vi "GotoWaypoint.vi"(7 "InhibitIn":bool, 8 "CurrentSteerAngle":dbl, 9 "WhatAroundMe? Clean":cluster{"T":dbl, "Range":dbl, "Bearing":dbl}[](array[cluster]), 10 "WhereAmI? Clean":T3, 11 "MDF In":T2(array[cluster])) -> (0 "BehCom":T1(ring), 1 "MDF Out":T2(array[cluster]), 2 "ActCommand":dbl[](array[numeric]), 4 "InhibitOut":bool, 5 "Vel":dbl, 6 "SteerAngle":dbl)   [LabVIEW 2012]
doc: "This subVI contains the Forebrain Goto Waypoint behaviors. Its inputs are the outputs of thewhat and where SENSE processes, theMission efinition Filet, a suppression value from another co-brahvior and an inhibit signal to turn the behavior off. The outputs are a 90 element steering array and a suppression value to diminish the output of co-behaviors.\n\nIt is designed to work with a 90 element behavior arbiter."
uses:
  <vilib>/Analysis/1siggen.llb/Ramp Pattern by Samples.vi
  <vilib>/gmath/statdist.llb/Normal PDF.vi
  <vilib>/gmath/NI_Gmath.lvlib
  <vilib>/Analysis/NI_AALBase.lvlib
panel:
  out "loop index":i32
  in  "HowAmI? Clean":cluster{"T":dbl, "Battery":dbl, "Temp":dbl}
  # "This VI contains the go to waypoint behavior  at the Forebrain level"
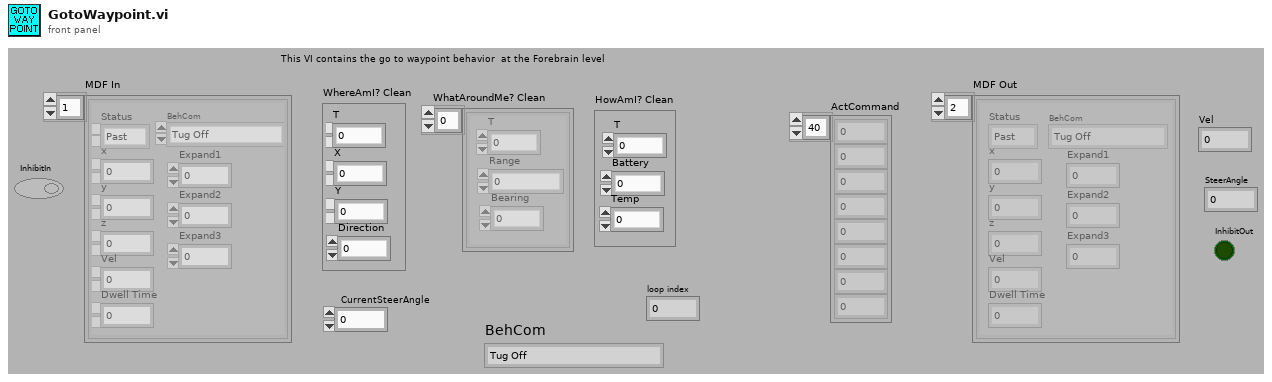
[diagram p1: front panel]
types:
  T1 = enum16{"Tug Off", "Manual Mode", "Goto WayPoint", "Back Up", "Circle", "Left Wall Follow", "Right Wall Follow", "Hunt"}
  T2 = cluster{"Status":enum16{"Past", "Current", "Future"}, "x":dbl, "y":dbl, "z":dbl, "Vel":dbl, "Dwell Time":dbl, "BehCom":enum16{"Tug Off", "Manual Mode", "Goto WayPoint", "Back Up", "Circle", "Left Wall Follow", "Right Wall Follow", "Hunt"}, "Expand1":dbl, "Expand2":dbl, "Expand3":dbl}[]
  T3 = cluster{"T":dbl, "X":dbl, "Y":dbl, "Direction":dbl}
  T4 = cluster{"Status":enum16{"Past", "Current", "Future"}, "x":dbl, "y":dbl, "z":dbl, "Vel":dbl, "Dwell Time":dbl, "BehCom":enum16{"Tug Off", "Manual Mode", "Goto WayPoint", "Back Up", "Circle", "Left Wall Follow", "Right Wall Follow", "Hunt"}, "Expand1":dbl, "Expand2":dbl, "Expand3":dbl}
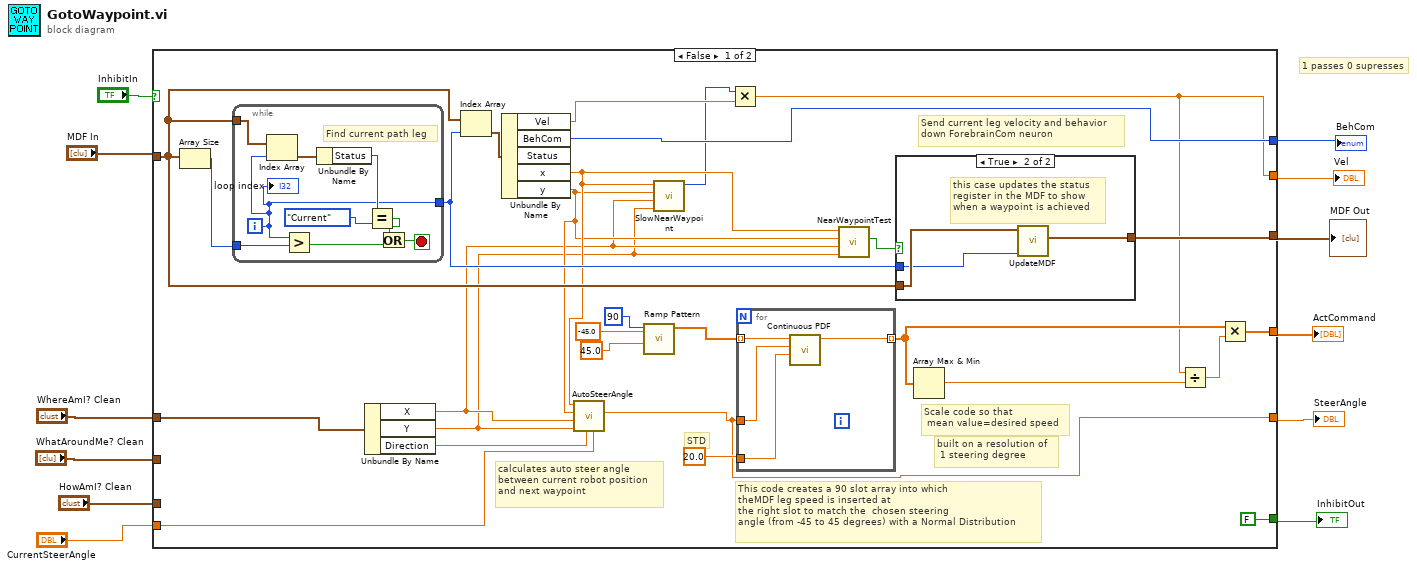
[diagram p0: block diagram]
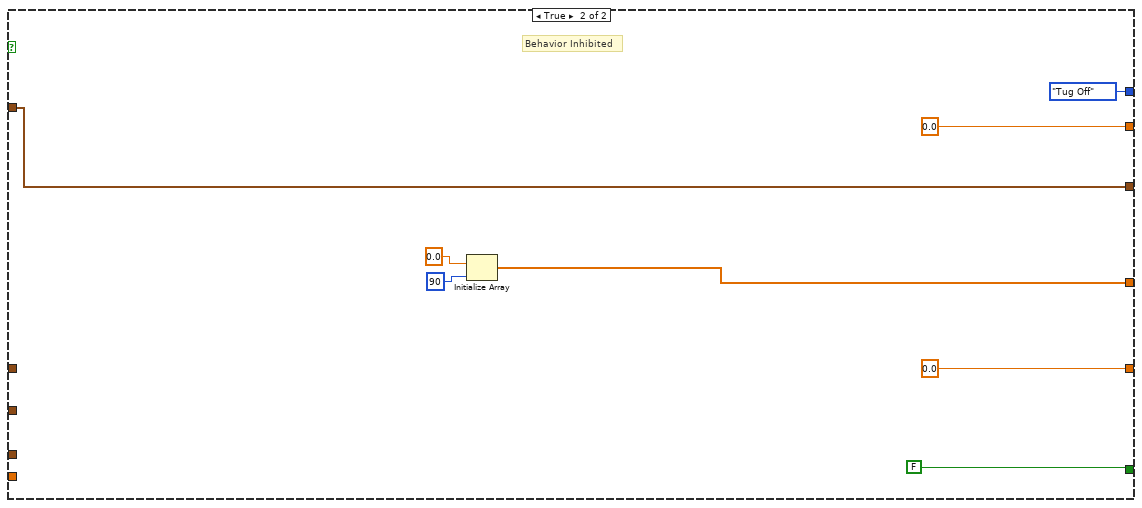
[diagram p3: hidden frame]
diagram:
  # "1 passes 0 supresses"
  n1 = case shown="False" "InhibitIn" {
    tunnel: "WhatAroundMe? Clean" -> [_ _]
    tunnel: "WhereAmI? Clean" -> [w38 _]
    tunnel: "HowAmI? Clean" -> [_ _]
    tunnel: [w28 w64] -> w7
    tunnel: [FALSE ("InhibitOut") FALSE ("InhibitOut")] -> w8
    tunnel: "MDF In" -> [w25 w61]
    tunnel: [w24 w61] -> w5
    tunnel: [w14 0.0 ("Vel")] -> w4
    tunnel: [w22 0.0 ("SteerAngle")] -> w3
    tunnel: "CurrentSteerAngle" -> [w21 _]
    tunnel: [w16 T1."Tug Off" ("BehCom")] -> w1
    frame False {
      # "Send current leg velocity and behavior\ndown ForebrainCom neuron"
      # "calculates auto steer angle\nbetween current robot position\nand next waypoint"
      # "built on a resolution of\n 1 steering degree"
      # "Scale code so that\n mean value=desired speed"
      # "STD"
      # "This code creates a 90 slot array into which\ntheMDF leg speed is inserted at\nthe right slot to match the  chosen steering\nangle (from -45 to 45 degrees) with a Normal Distribution"
      n2 = Array Size(array=w25) -> (size(s)=w39:i32)
      n3 = while {
        tunnel: w39 -> [w57]
        tunnel: w25 -> [w54]
        tunnel: [w49] -> w23
        i -> [w49]
        stop <- w56 stop-if-true
        # "Find current path leg"
        n4 = Index Array "Index Array"(array=w54, index=w49) -> (element=w51:T4)
        n5 = Greater?(x=w49, y=w57) -> (0:w55:bool)
        n6 = Unbundle By Name(w51) -> ("Status"=w52:enum16{"Past", "Current", "Future"})
        n7 = Equal?(x=w52, y=enum16{"Past", "Current", "Future"}."Current") -> (x = y?=w53:bool)
        n8 = Or(x=w53, y=w55) -> (x .or. y?=w56:bool)
        "loop index" <- w49
      }
      n9 = Unbundle By Name(w38) -> ("X"=w18:dbl, "Y"=w17:dbl, "Direction"=w27:dbl)
      n10 = Index Array "Index Array"(array=w25, index=w23) -> (element=w37:T4)
      n11 = Unbundle By Name(w37) -> ("Vel"=w15:dbl, "BehCom"=w16:T1, "x"=w20:dbl, "y"=w19:dbl)  [unwired: 1 out]
      n12 = call "AutoSteerAngle.vi"("CurrentSteerAngle"=w21, "CurrentDirection"=w27, "Ycurrent"=w17, "Xcurrent"=w18, "Ywaypoint"=w19, "Xwaypoint"=w20) -> ("NewSteerAngle"=w22:dbl)  [unwired: 5 in]
      n13 = call-poly <vilib>:"Ramp Pattern.vi"("start"=45.0, "end"=-45.0 ("end (Normal)"), "samples"=90) -> ("Ramp Pattern"=w31:dbl[])  [unwired: 7 in, 1 out]
      n14 = call "SlowNearWaypoint.vi"("Yrobot"=w17, "Xrobot"=w18, "Ywaypoint"=w19, "Xwaypoiny"=w20) -> ("SpeedDecrease"=w13:i32)  [unwired: 7 in]
      n15 = Multiply(x=w13, y=w15) -> (x*y=w14:dbl)
      n16 = for {
        tunnel: w31 -> [w48] mode=indexing
        tunnel: 20.0 ("std (Normal)") -> [w47]
        tunnel: [w46] -> w35 mode=indexing
        tunnel: w22 -> [w45]
        n17 = call-poly <vilib>:"Continuous PDF.vi"("std"=w47, "mean"=w45, "x"=w48) -> ("pdf(x)"=w46:dbl)  [unwired: 7 in, 1 out]
      }
      n18 = call "NearWaypointTest.vi"("Yrobot"=w17, "Xrobot"=w18, "Ywaypoint"=w19, "Xwaypoiny"=w20) -> ("AtWaypoint"=w26:bool)  [unwired: 7 in]
      n19 = case shown="True" w26 {
        tunnel: w25 -> [w41 w44]
        tunnel: [w41 w42] -> w24
        tunnel: w23 -> [_ w43]
        frame False {
          # "robot not near waypoint\npass MDF through unaltered"
        }
        frame True {
          # "this case updates the status\nregister in the MDF to show \nwhen a waypoint is achieved"
          n20 = call "UpdateMDF.vi"("Index"=w43, "MDF_In"=w44) -> ("MDF_Out"=w42:T2)  [unwired: 9 in]
        }
      }
      n21 = Array Max & Min(array=w35) -> (max value=w33:dbl)  [unwired: 3 out]
      n22 = Divide(x=w14, y=w33) -> (x/y=w34:dbl)
      n23 = Multiply(x=w35, y=w34) -> (x*y=w28:dbl[])
    }
    frame True {
      # "Behavior Inhibited"
      n24 = Initialize Array "Initialize Array"(0.0 ("element"), 90 ("dimension size")) -> (w64:dbl[])
    }
  }
  "ActCommand" <- w7
  "InhibitOut" <- w8
  "MDF Out" <- w5
  "Vel" <- w4
  "SteerAngle" <- w3
  "BehCom" <- w1
